vi "Read Analogue.vi"(8 "error in (no error)":errorcluster, 11 "Voltage Input in":refnum<class "Hioki BT4560B.lvclass">) -> (0 "error out":errorcluster, 2 "Measurement":dbl format="%.5f", 3 "Voltage Input out":refnum<class "Hioki BT4560B.lvclass">)   [LabVIEW 2021, in "Concrete.lvlib" / "Hioki BT4560B.lvclass"]
uses:
  Hioki BT4560B.lvclass
  Hioki BT4560B.lvclass/Hioki BT4560B.ctl
  Harware Abstraction/AnalogIO/AIO.lvclass
  <instrlib>/HIOKI BT4560/HIOKI BT4560.lvlib
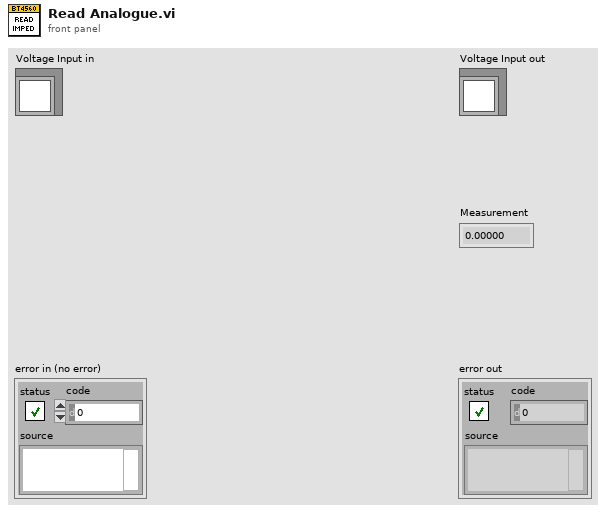
[diagram p1: front panel]
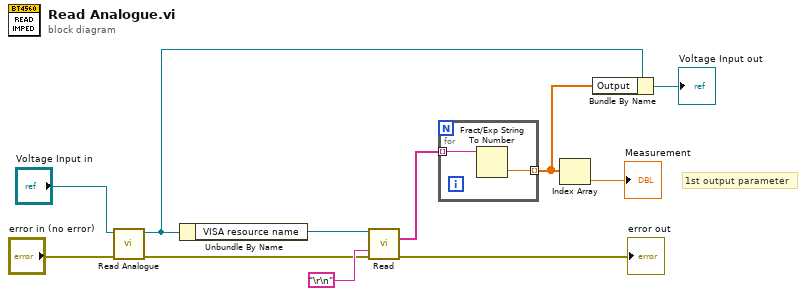
[diagram p0: block diagram]
diagram:
  # "1st output parameter"
  n1 = call-parent "Read Analogue.vi"("error in (no error)"="error in (no error)", "PS in"="Voltage Input in") -> ("error out"=w6:errorcluster, "PS out"=w3:refnum<class "Hioki BT4560B.lvclass">)  [unwired: 7 in, 1 out]
  n2 = Unbundle By Name(w3) -> ("VISA resource name"=w7:refnum<visa-resource-name>)
  n3 = call <instrlib>:"Read.vi"("VISA session"=w7, "Terminator"="\r\n", "error in (no error)"=w6) -> ("Output Str"=w9:string[], "error out"=→"error out":errorcluster)  [unwired: 9 in, 2 out]
  n4 = for {
    tunnel: w9 -> [w13] mode=indexing
    tunnel: [w12] -> w2 mode=indexing
    n5 = Fract/Exp String To Number(string=w13) -> (number=w12:dbl)  [unwired: 3 in, 1 out]
  }
  n6 = Index Array(array=w2) -> (element=→"Measurement":dbl)  [unwired: 1 in]
  n7 = Bundle By Name(cluster=w3, "Output"=w2) -> (→"Voltage Input out":refnum<class "Hioki BT4560B.lvclass">)
